vi "VS-Heart Rate From ABR.vi"(0 "Settings":T1, 9 "Sampling Rate (Hz)":dbl=10000.0) -> (6 "Heart Rate (bpm)":dbl format="%.1f", 10 "XY Graph":cluster{"Array":dbl[], "Filtered X":dbl[]}[](graph), 14 "Raw waveform":dbl[](array[numeric]), 15 "error out":errorcluster)   [LabVIEW 2020]
uses:
  Typedefs/PhysMon-HR From EKG Settings.ctl
panel:
  # "Measuring heart rate...."
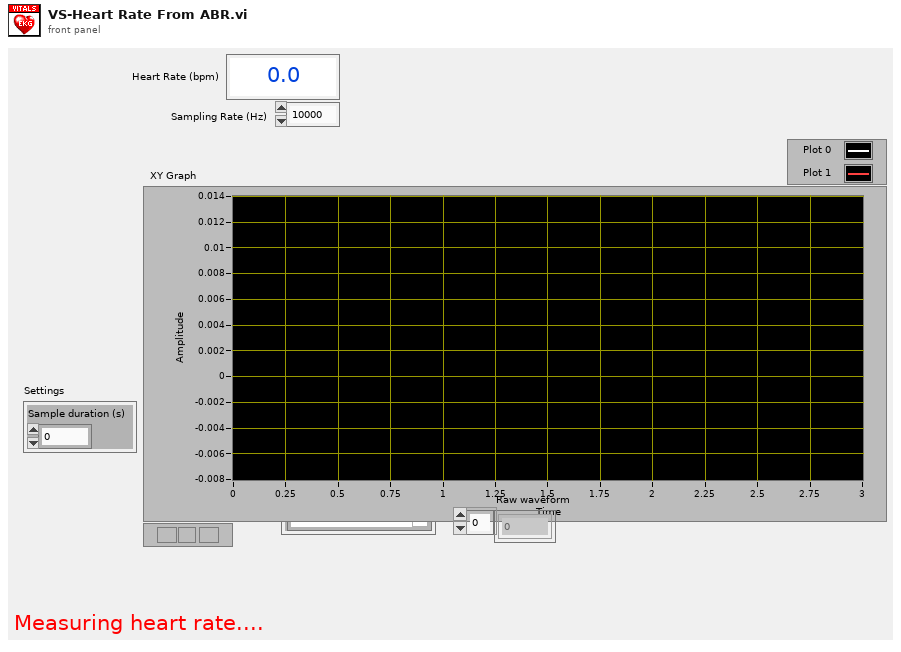
[diagram p1: front panel]
types:
  T1 = typedef "PhysMon-HR From EKG Settings.ctl" = cluster{"Sample duration (s)":dbl}
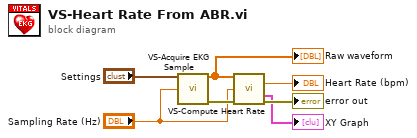
[diagram p0: block diagram]
diagram:
  n1 = call "VS-Acquire EKG Sample.vi"("Settings"="Settings", "Sampling Rate (Hz)"="Sampling Rate (Hz)") -> ("Waveform"=w4:dbl[], "error out"=w6:errorcluster)  [unwired: 12 in]
  "Raw waveform" <- w4
  n2 = call "VS-Compute Heart Rate.vi"("ECG"=w4, "Sampling Rate (Hz)"="Sampling Rate (Hz)", "error in (no error)"=w6) -> ("Heart Rate (bpm)"=→"Heart Rate (bpm)":dbl, "XY Graph"=→"XY Graph":cluster{"Array":dbl[], "Filtered X":dbl[]}[], "error out"=→"error out":errorcluster)  [unwired: 10 in]
